vi "ASrreglo3disp.vi"(4 "datos":dbl[][](array[numeric]), 5 "disp. 3":i32, 6 "disp. 2":i32, 7 "disp. 1":i32, 10 "output array 2":dbl[][][][][](array[numeric])) -> (2 "output array":dbl[][][][][](array[numeric]))   [LabVIEW 2016]
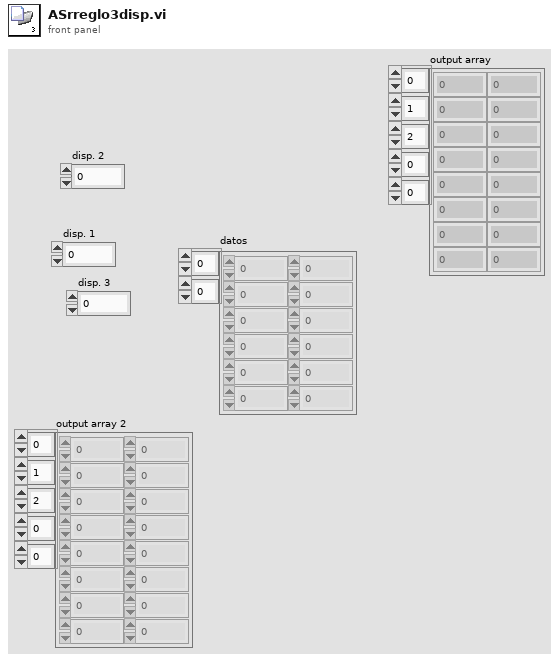
[diagram p1: front panel]
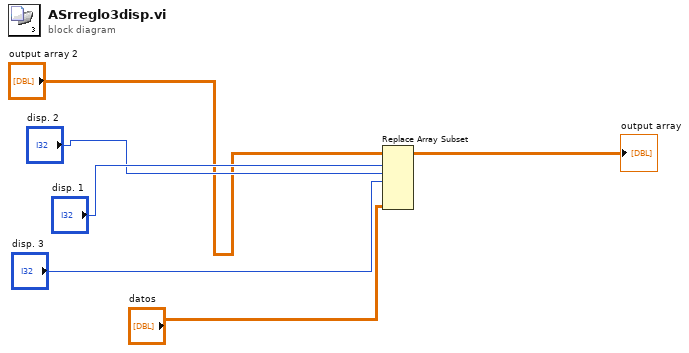
[diagram p0: block diagram]
diagram:
  n1 = Replace Array Subset(array="output array 2", new element="datos", index (dim 0)="disp. 1", index (dim 1)="disp. 2", index (dim 2)="disp. 3") -> (→"output array":dbl[][][][][])  [unwired: 2 in]
